vi "Destroy.vi"(0 "reference in":refnum<class "excelFile.lvclass">, 5 "error in (no error)":errorcluster) -> (14 "reference out":refnum<class "excelFile.lvclass">, 19 "error out":errorcluster)   [LabVIEW 2015, in "excelFile.lvclass"]
doc: "Destructor."
uses:
  excelFile.lvclass
  <vilib>/addons/_AddQ/G#Object/G#Object.lvclass
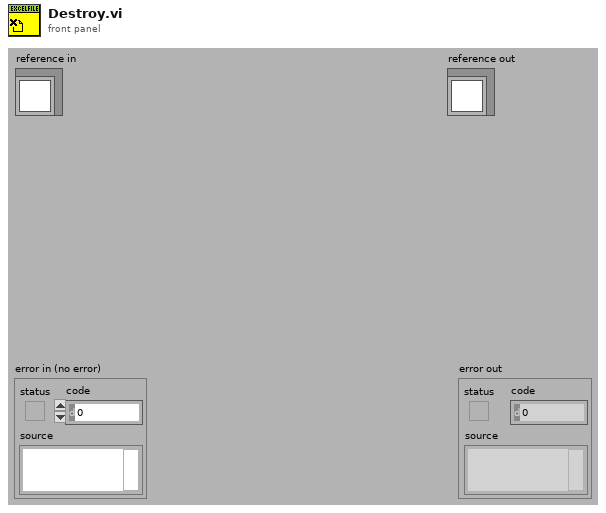
[diagram p1: front panel]
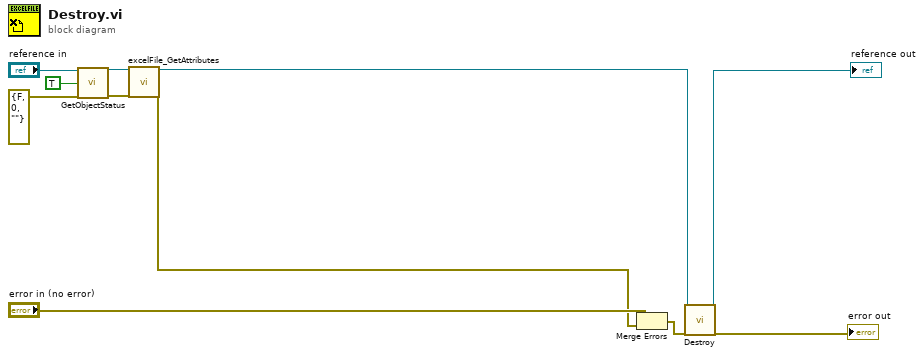
[diagram p0: block diagram]
diagram:
  n1 = call-dynamic "GetObjectStatus.vi"("reference in"="reference in", "simple info (F)"=TRUE ("simple info"), "error in (no error)"=errorcluster {"status"=FALSE, "code"=0, "source"=""}) -> ("reference out"=w5:refnum<class "excelFile.lvclass">, "error out"=w6:errorcluster)  [unwired: 5 in, 10 out]
  n2 = call "excelFile_GetAttributes.vi"("reference in"=w5, "error in (no error)"=w6) -> ("reference out"=w4:refnum<class "excelFile.lvclass">, "error out"=w1:errorcluster)  [unwired: 14 in, 2 out]
  n3 = Merge Errors("error in (no error)", w1) -> (w10:errorcluster)
  n4 = call-parent "Destroy.vi"("reference in"=w4, "error in (no error)"=w10) -> ("reference out"=→"reference out":refnum<class "excelFile.lvclass">, "error out"=→"error out":errorcluster)  [unwired: 16 in]
